vi "GaussianRowLocation.vi"(11 "Comments":string) -> (3 "RowXPosition":dbl)   [LabVIEW 2011]
panel:
  out "ChannelStrings":string[](array[string])
  out "error out":errorcluster
  in  "error in":errorcluster
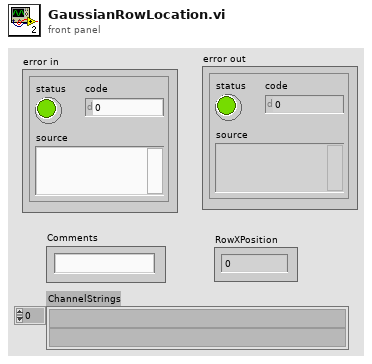
[diagram p1: front panel]
types:
  T1 = enum16{"open", "replace", "create", "open or create", "replace or create", "replace or create with confirmation"}
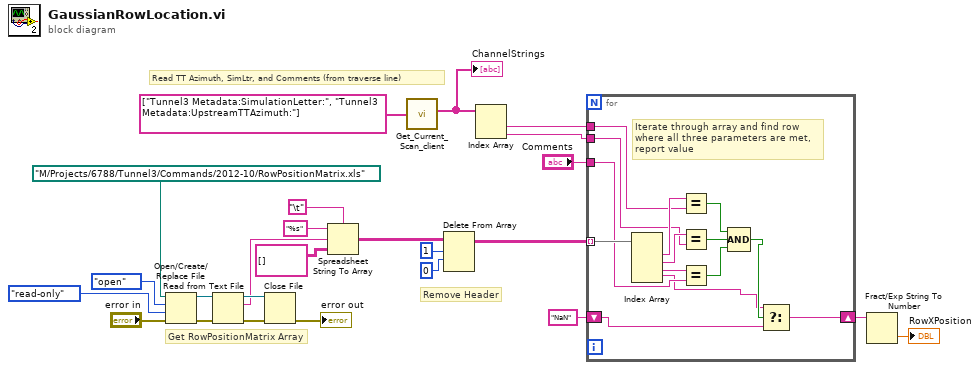
[diagram p0: block diagram]
diagram:
  # "Read TT Azimuth, SimLtr, and Comments (from traverse line)"
  # "Get RowPositionMatrix Array"
  # "Remove Header"
  n1 = Open/Create/Replace File(file path (use dialog)=path "M:/Projects/6788/Tunnel3/Commands/2012-10/RowPositionMatrix.xls", error in="error in", operation (0:open)=T1."open", access (0:read/write)=enum16{"read/write", "read-only", "write-only"}."read-only") -> (refnum out=w19:refnum<file>, error out=w20:errorcluster)  [unwired: 2 in, 1 out]
  n2 = Read from Text File(file (use dialog)=w19, error in=w20) -> (refnum out=w17:refnum<file>, text=w15:string, error out=w18:errorcluster)  [unwired: 2 in, 1 out]
  n3 = Close File(refnum=w17, error in=w18) -> (error out=→"error out":errorcluster)  [unwired: 1 out]
  n4 = Spreadsheet String To Array(delimiter (Tab)="\t", format string="%s", spreadsheet string=w15, array type (2D Dbl)=string[][] []) -> (array=w11:string[][])
  n5 = call "Get_Current_Scan_client.vi"("ADAM Ch Names"=string[] ["Tunnel3 Metadata:SimulationLetter:", "Tunnel3 Metadata:UpstreamTTAzimuth:"]) -> ("String values"=w4:string[])  [unwired: 1 in, 2 out]
  "ChannelStrings" <- w4
  n6 = Delete From Array(array=w11, length=1, index (row)=0) -> (array with subset deleted=w8:string[][])  [unwired: 1 in, 1 out]
  n7 = Index Array(array=w4) -> (element #1=w6:string, element #2=w5:string)  [unwired: 2 in]
  n8 = for {
    tunnel: w8 -> [w39] mode=indexing
    tunnel: "Comments" -> [w33]
    tunnel: w6 -> [w37]
    tunnel: w5 -> [w35]
    shift-right: [w27] -> w1
    shift-left: "NaN" -> [w26]
    # "Iterate through array and find row where all three parameters are met, report value"
    n9 = Index Array(array=w39) -> (element #1=w38:string, element #2=w36:string, element #3=w34:string, element #4=w28:string)  [unwired: 4 in]
    n10 = Equal?(x=w38, y=w37) -> (x = y?=w32:bool)
    n11 = Equal?(x=w36, y=w35) -> (x = y?=w31:bool)
    n12 = Equal?(x=w34, y=w33) -> (x = y?=w30:bool)
    n13 = Compound Arithmetic op=AND(w32, w31, w30) -> (w29:bool)
    n14 = Select(t=w28, s=w29, f=w26) -> (s? t:f=w27:string)
  }
  n15 = Fract/Exp String To Number(string=w1) -> (number=→"RowXPosition":dbl)  [unwired: 3 in, 1 out]
